vi "Mätprogram.vi"(6 "Tidsfönster [s]":string="10", 8 "Mitt av hysteres [V]":string="2.0", 9 "Hysteresprocent [0|50|100]":string="100", 10 "Trigger slope [POS|NEG]":string="POS", 11 "GPIB Frekvensräknare":string="4") -> (2 "mätvärde":dbl)   [LabVIEW 2020]
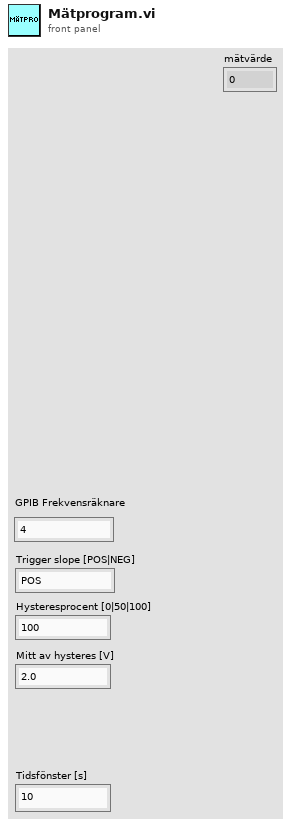
[diagram p1: front panel]
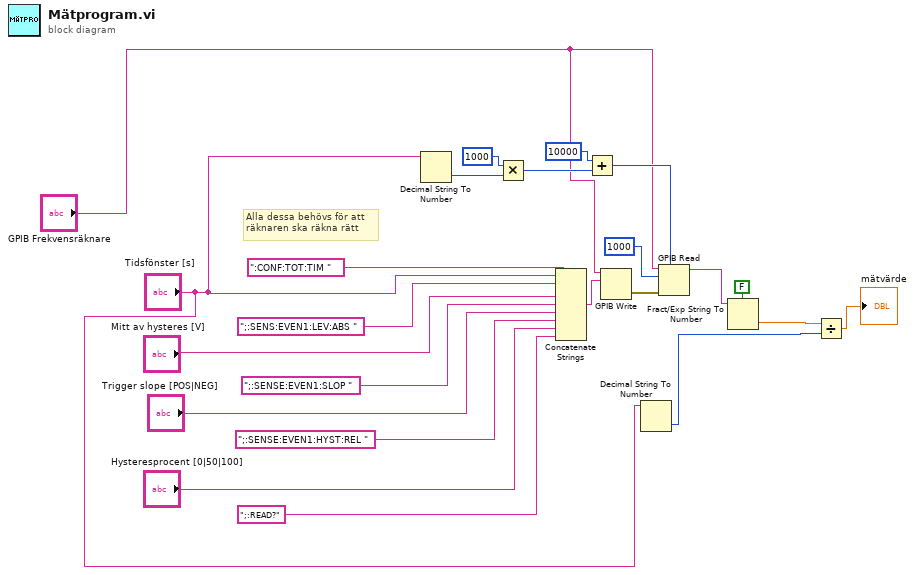
[diagram p0: block diagram]
diagram:
  # "Alla dessa behövs för att \nräknaren ska räkna rätt"
  n1 = Decimal String To Number(string="Tidsfönster [s]") -> (number=w15:i32)  [unwired: 2 in, 1 out]
  n2 = Multiply(x=1000, y=w15) -> (x*y=w17:i32)
  n3 = Concatenate Strings(":CONF:TOT:TIM " ("string"), "Tidsfönster [s]", ";:SENS:EVEN1:LEV:ABS " ("string"), "Mitt av hysteres [V]", ";:SENSE:EVEN1:SLOP " ("string"), "Trigger slope [POS|NEG]", ";:SENSE:EVEN1:HYST:REL " ("string"), "Hysteresprocent [0|50|100]", ";:READ?" ("string")) -> (w20:string)
  n4 = Add(x=10000, y=w17) -> (x+y=w21:i32)
  n5 = GPIB Write(0:"GPIB Frekvensräknare", 1:w20) -> (6:w23:errorcluster)  [unwired: 3 in, 1 out]
  n6 = Decimal String To Number(string="Tidsfönster [s]") -> (number=w3:i32)  [unwired: 2 in, 1 out]
  n7 = GPIB Read(0:"GPIB Frekvensräknare", 1:1000 ("byte count"), 3:w23, 4:w21) -> (5:w13:string)  [unwired: 1 in, 2 out]
  n8 = Fract/Exp String To Number(use system decimal point (T)=FALSE, string=w13) -> (number=w2:dbl)  [unwired: 2 in, 1 out]
  n9 = Divide(x=w2, y=w3) -> (x/y=→"mätvärde":dbl)
